vi "Assert In Range.vi"(3 "Execution time (s)":dbl=-1.0, 4 "Register with caller test (F)":bool, 5 "Assert Only? (F)":bool, 6 "error code (1)":i32=1, 7 "Label (\"\")":string, 8 "error in (no error)":errorcluster, 9 "Lower Limit":ext, 10 "Upper Limit":ext, 11 "X":ext) -> (0 "error out":errorcluster, 2 "Properties.Assert":refnum<class "Properties.Assert.lvclass">)   [LabVIEW 2013, in "Caraya.lvlib" / "Assert.lvclass"]
doc: "Asserts that <B>X</B> is between <B>upper limit</B> and <B>lower limit</B>."
uses:
  Assert.lvclass
  Properties.Assert/Properties.Assert.lvclass
  Properties/Properties.lvclass
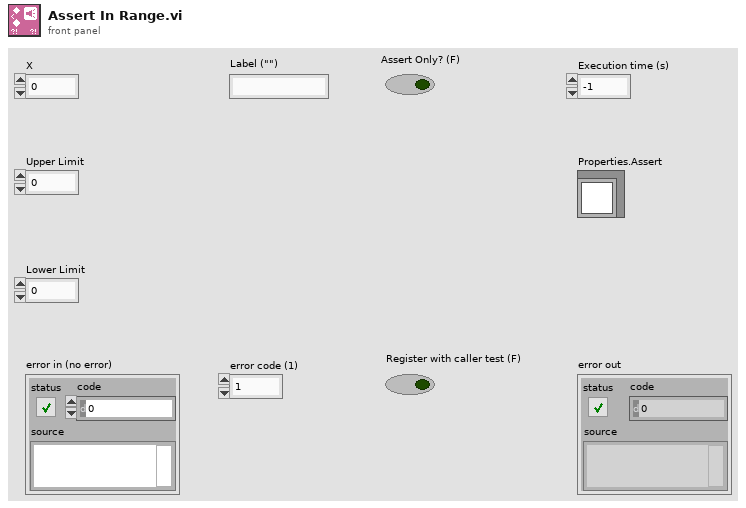
[diagram p1: front panel]
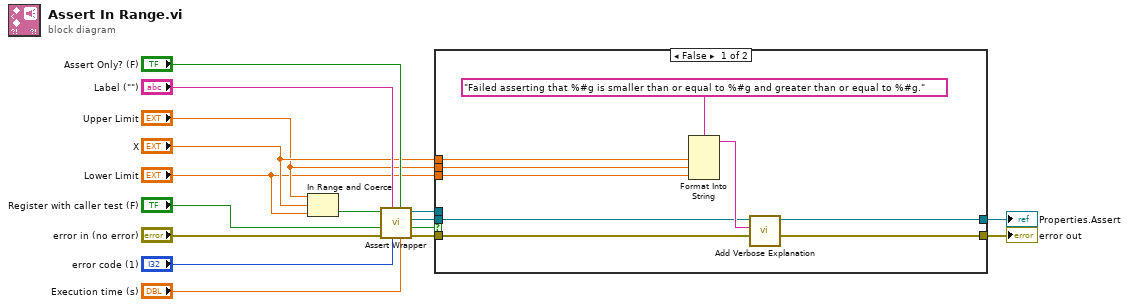
[diagram p0: block diagram]
diagram:
  n1 = In Range and Coerce(upper limit="Upper Limit", x="X", lower limit="Lower Limit") -> (In Range?=w4:bool)  [unwired: 1 out]
  n2 = call "Assert Wrapper.vi"("Execution time (s)"="Execution time (s)", "Assert Only? (F)"="Assert Only? (F)", "error code (1)"="error code (1)", "Label"="Label (\"\")", "error in (no error)"="error in (no error)", "Register with caller test (F)"="Register with caller test (F)", "Assert?"=w4) -> ("error out"=w7:errorcluster, "Verbose"=w11:bool, "Properties.Assert"=w9:refnum<class "Properties.Assert.lvclass">, "Assert out"=w10:refnum<class "Assert.lvclass">)  [unwired: 1 in]
  n3 = case shown="False" w11 {
    tunnel: w10 -> [_ _]
    tunnel: w9 -> [w22 w27]
    tunnel: [w24 w26] -> w8
    tunnel: w7 -> [w25 w26]
    tunnel: [w21 w27] -> w6
    tunnel: "X" -> [w19 _]
    tunnel: "Upper Limit" -> [w18 _]
    tunnel: "Lower Limit" -> [w17 _]
    frame False {
      n4 = Format Into String(format string="Failed asserting that %#g is smaller than or equal to %#g and greater than or equal to %#g.", w19, w18, w17) -> (resulting string=w23:string)  [unwired: 2 in, 1 out]
      n5 = call "Add Verbose Explanation.vi"("error in (no error)"=w25, "Verbose Explanation"=w23, "Properties"=w22) -> ("error out"=w24:errorcluster, "Properties"=w21:refnum<class "Properties.Assert.lvclass">)  [unwired: 7 in]
    }
    frame True {
    }
  }
  "error out" <- w8
  "Properties.Assert" <- w6
